vi "CohortSet.vi"(6 "Set COR Tag":string, 7 "Set Electrodes":sgl[](array[numeric]), 8 "error in (no error)":errorcluster, 9 "Set Pulse Width":sgl, 10 "Set Pulse Frequency":sgl format="%6.2f") -> (0 "error out":errorcluster, 3 "Cohort out":refnum<class "Cohort.lvclass">)   [LabVIEW 2012, in "Cohort.lvclass"]
uses:
  Cohort.lvclass
  Cohort.lvclass/Cohort.ctl
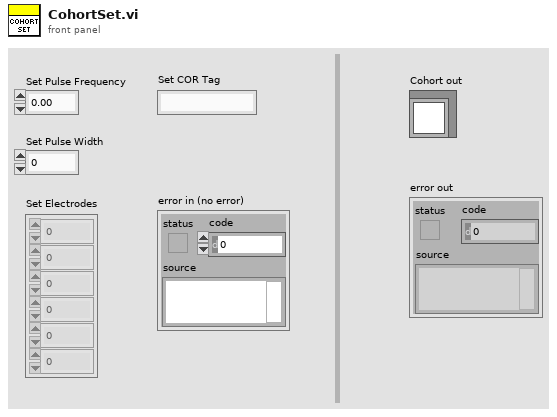
[diagram p1: front panel]
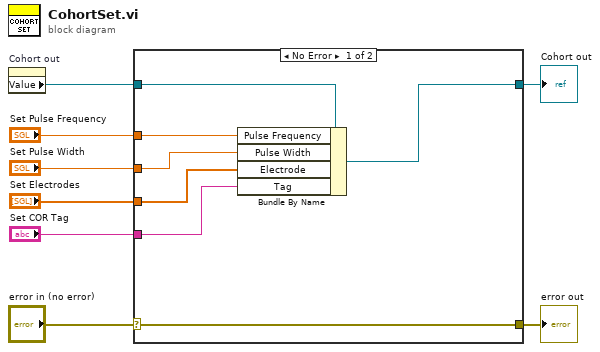
[diagram p0: block diagram]
diagram:
  n1 = property on="Cohort out" class="LVClassControl (strict)"() -> ("Value"=w2:refnum<class "Cohort.lvclass">)  [unwired: 2 in, 2 out]
  n2 = case shown="No Error" "error in (no error)" {
    selector: "error in (no error)" -> [w15 w16]
    tunnel: [w15 w16] -> w7
    tunnel: [w13 w17] -> w6
    tunnel: w2 -> [w14 w17]
    tunnel: "Set Pulse Frequency" -> [w12 _]
    tunnel: "Set Pulse Width" -> [w11 _]
    tunnel: "Set Electrodes" -> [w10 _]
    tunnel: "Set COR Tag" -> [w9 _]
    frame No Error {
      n3 = Bundle By Name(cluster=w14, "Pulse Frequency"=w12, "Pulse Width"=w11, "Electrode"=w10, "Tag"=w9) -> (w13:refnum<class "Cohort.lvclass">)
    }
    frame Error {
    }
  }
  "error out" <- w7
  "Cohort out" <- w6
